vi "Support_Amalgamation.vi"(8 "error in (no error)":errorcluster, 11 "AB_Dest_App in":refnum<class "AB_Dest_App.lvclass">) -> (0 "error out":errorcluster, 3 "Supports amalgamations?":bool)   [LabVIEW 2020, in "AB_Dest_App.lvclass"]
uses:
  <vilib>/AppBuilder/AB_Classes/Destination/Dest_Application/AB_Dest_App.lvclass
  e:/builds/penguin/labview/branches/2020/dev/dist/vi.lib/AppBuilder/AB_Classes/Destination/AB_Destination.lvclass
  <vilib>/AppBuilder/AB_Classes/Destination/AB_Destination.lvclass
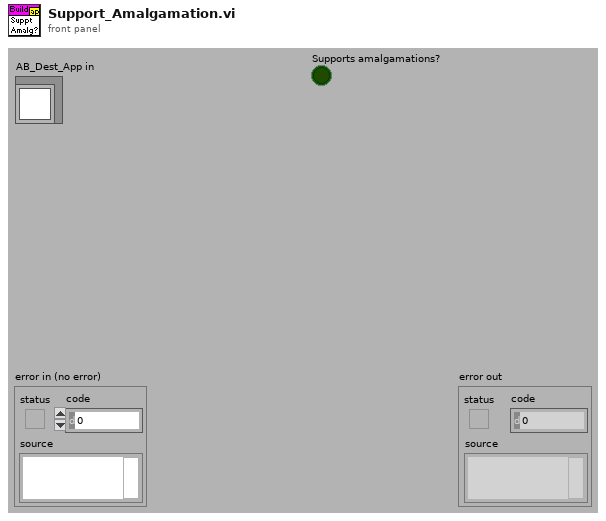
[diagram p1: front panel]
types:
  T1 = typedef "AB_Destination.ctl" = cluster{"destName":string, "path":path, "libraryName":string, "preserveHierarchy":bool, "eng_inBuild":bool, "eng_libraryReference":refnum<vi>, "eng_restictAddToNewLibrary":bool}
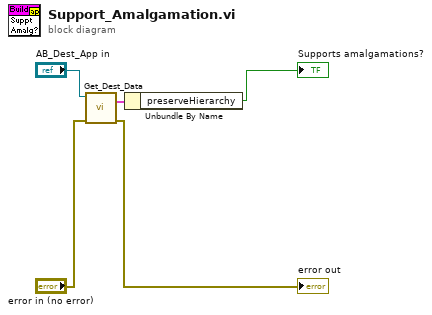
[diagram p0: block diagram]
diagram:
  n1 = call <vilib>:"Get_Dest_Data.vi"("error in (no error)"="error in (no error)", "Class in"="AB_Dest_App in") -> ("error out"=→"error out":errorcluster, "destName"=w3:T1)  [unwired: 8 out]
  n2 = Unbundle By Name(w3) -> ("preserveHierarchy"=→"Supports amalgamations?":bool)
